vi "2013_01_17 Quality Main.vi"() -> ()   [LabVIEW 2011]
uses:
  <vilib>/DAQmx/write.llb/DAQmx Write (Counter Time 1Chan 1Samp).vi
  <vilib>/DAQmx/read.llb/DAQmx Read (Analog 1D Wfm NChan NSamp).vi
  Quality Type Def.ctl
panel:
  out "position mode":i32
  out "samples available":i32
  in  "Choose Lead":dbl=1.0 min=1.0 max=2.0 step=1.0
  out "XY Graph 2":cluster{"Array":dbl[], "Array":dbl[]}[](graph)
  out "Single Motor 2":waveform(dbl)[](graph)
  in  "Waveform":bool
  out "XY Graph":cluster{"Array":dbl[], "Array":dbl[]}(graph)
  out "error out":errorcluster
  in  "File Path":path=path "Durability/.lvm"
  in  "Motor 1":T1 {"ESC Efficiency" format="%#_3g%%"; "Supply Power (W)" format="%.3g"; "Mechanical Power (W)" format="%.3g"; "Motor Efficiency" format="%#_3g%%"; "Electrical Power (W)" format="%.3g"; "Torque (mNm)" format="%.3g"; "Elapsed Time" format="%<%H:%M:%S>t"; "Supply (V)" format="%.2f"; "RPM" scale=0.0..60000.0}
  out "loop time (ms)":u32
  in  "stop":bool
  in  "PWM 1":dbl(slide) min=0.0 max=100.0 step=5.0 scale=0.0..100.0
  # "Fail"
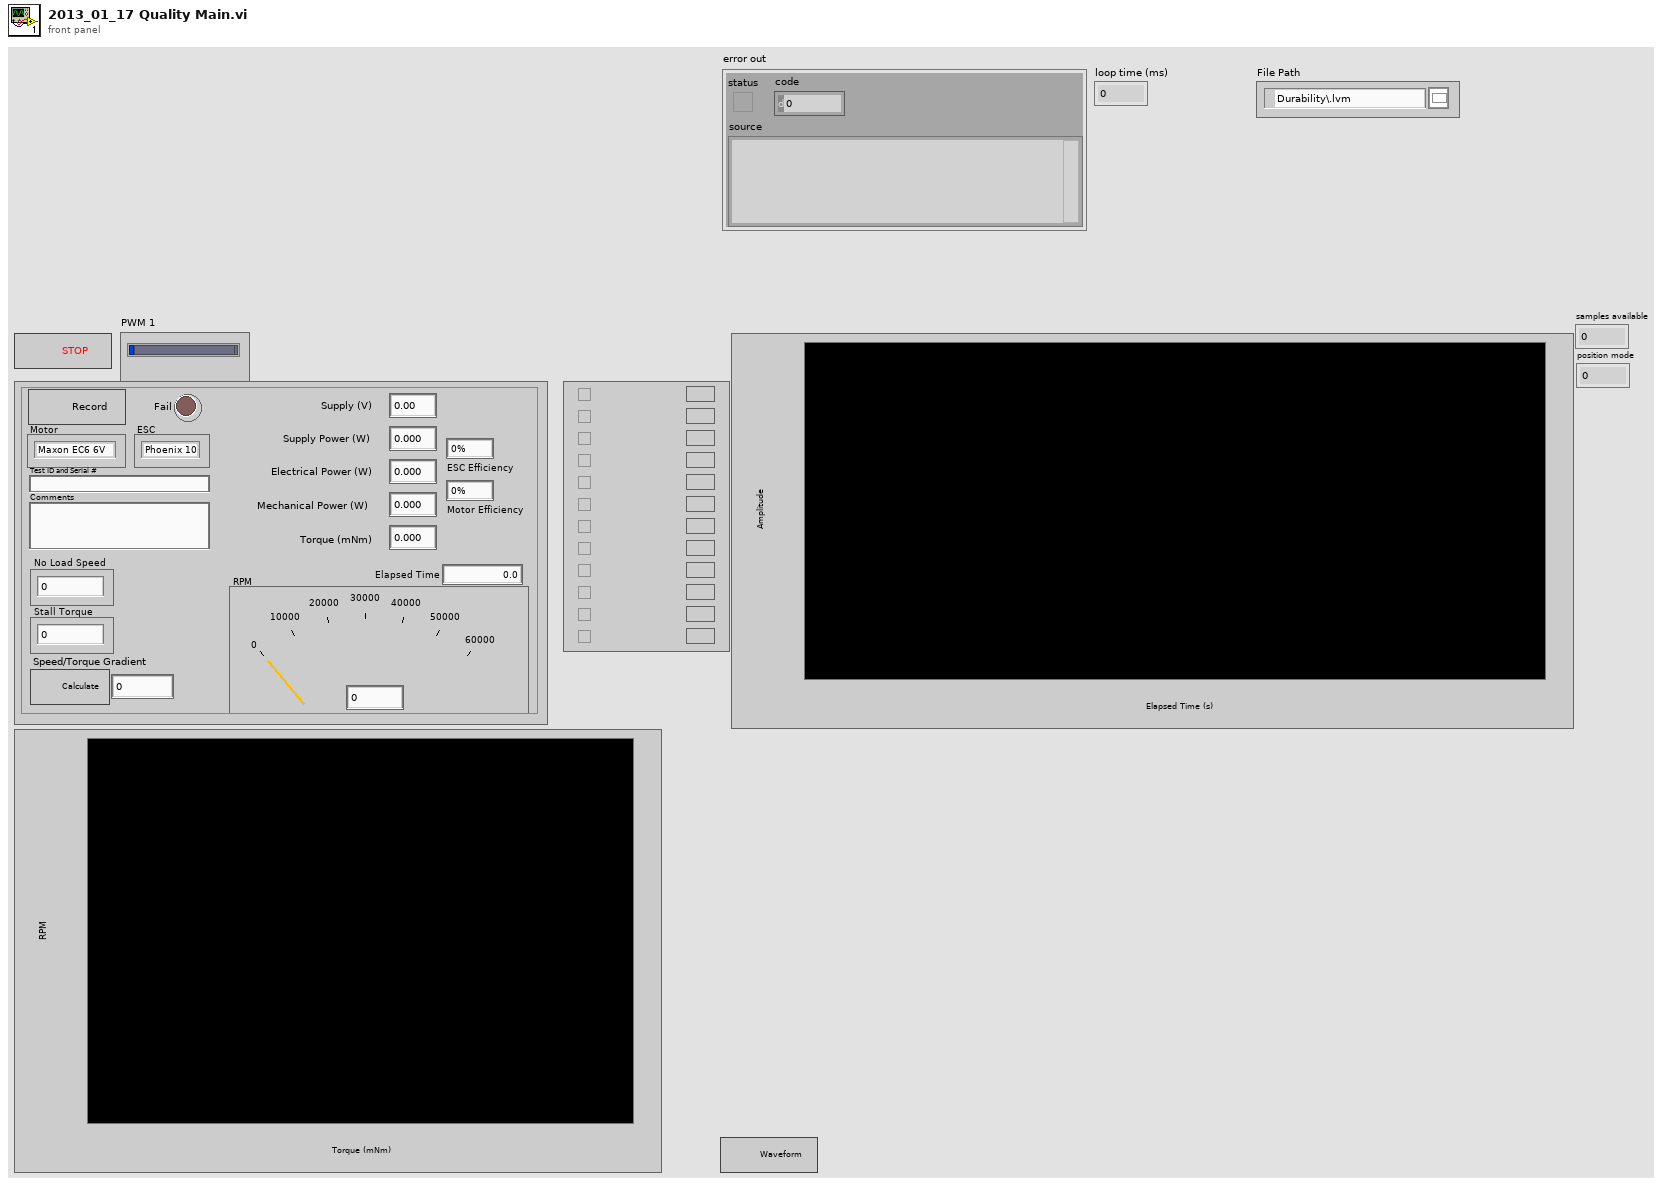
[diagram p1: front panel]
types:
  T1 = typedef "Quality Type Def.ctl" = cluster{"Enabled":bool, "Fail":bool, "RPM":u64, "Motor":enum16{"Maxon EC6 6V", "Maxon EC4 6V", "FH 0620 6V", "FH 0620 12V"}, "ESC":enum16{"Phoenix 10", "Maxon", "FH 1801"}, "Supply (V)":dbl, "Test ID and Serial #":string, "Comments":string, "Elapsed Time":dbl, "Counter":dbl, "Torque (mNm)":dbl, "Electrical Power (W)":dbl, "Motor Efficiency":dbl, "Mechanical Power (W)":dbl, "Supply Power (W)":dbl, "ESC Efficiency":dbl, "No Load Speed":u32, "Stall Torque":dbl, "Speed/Torque Gradient":u32, "Calcul":bool}
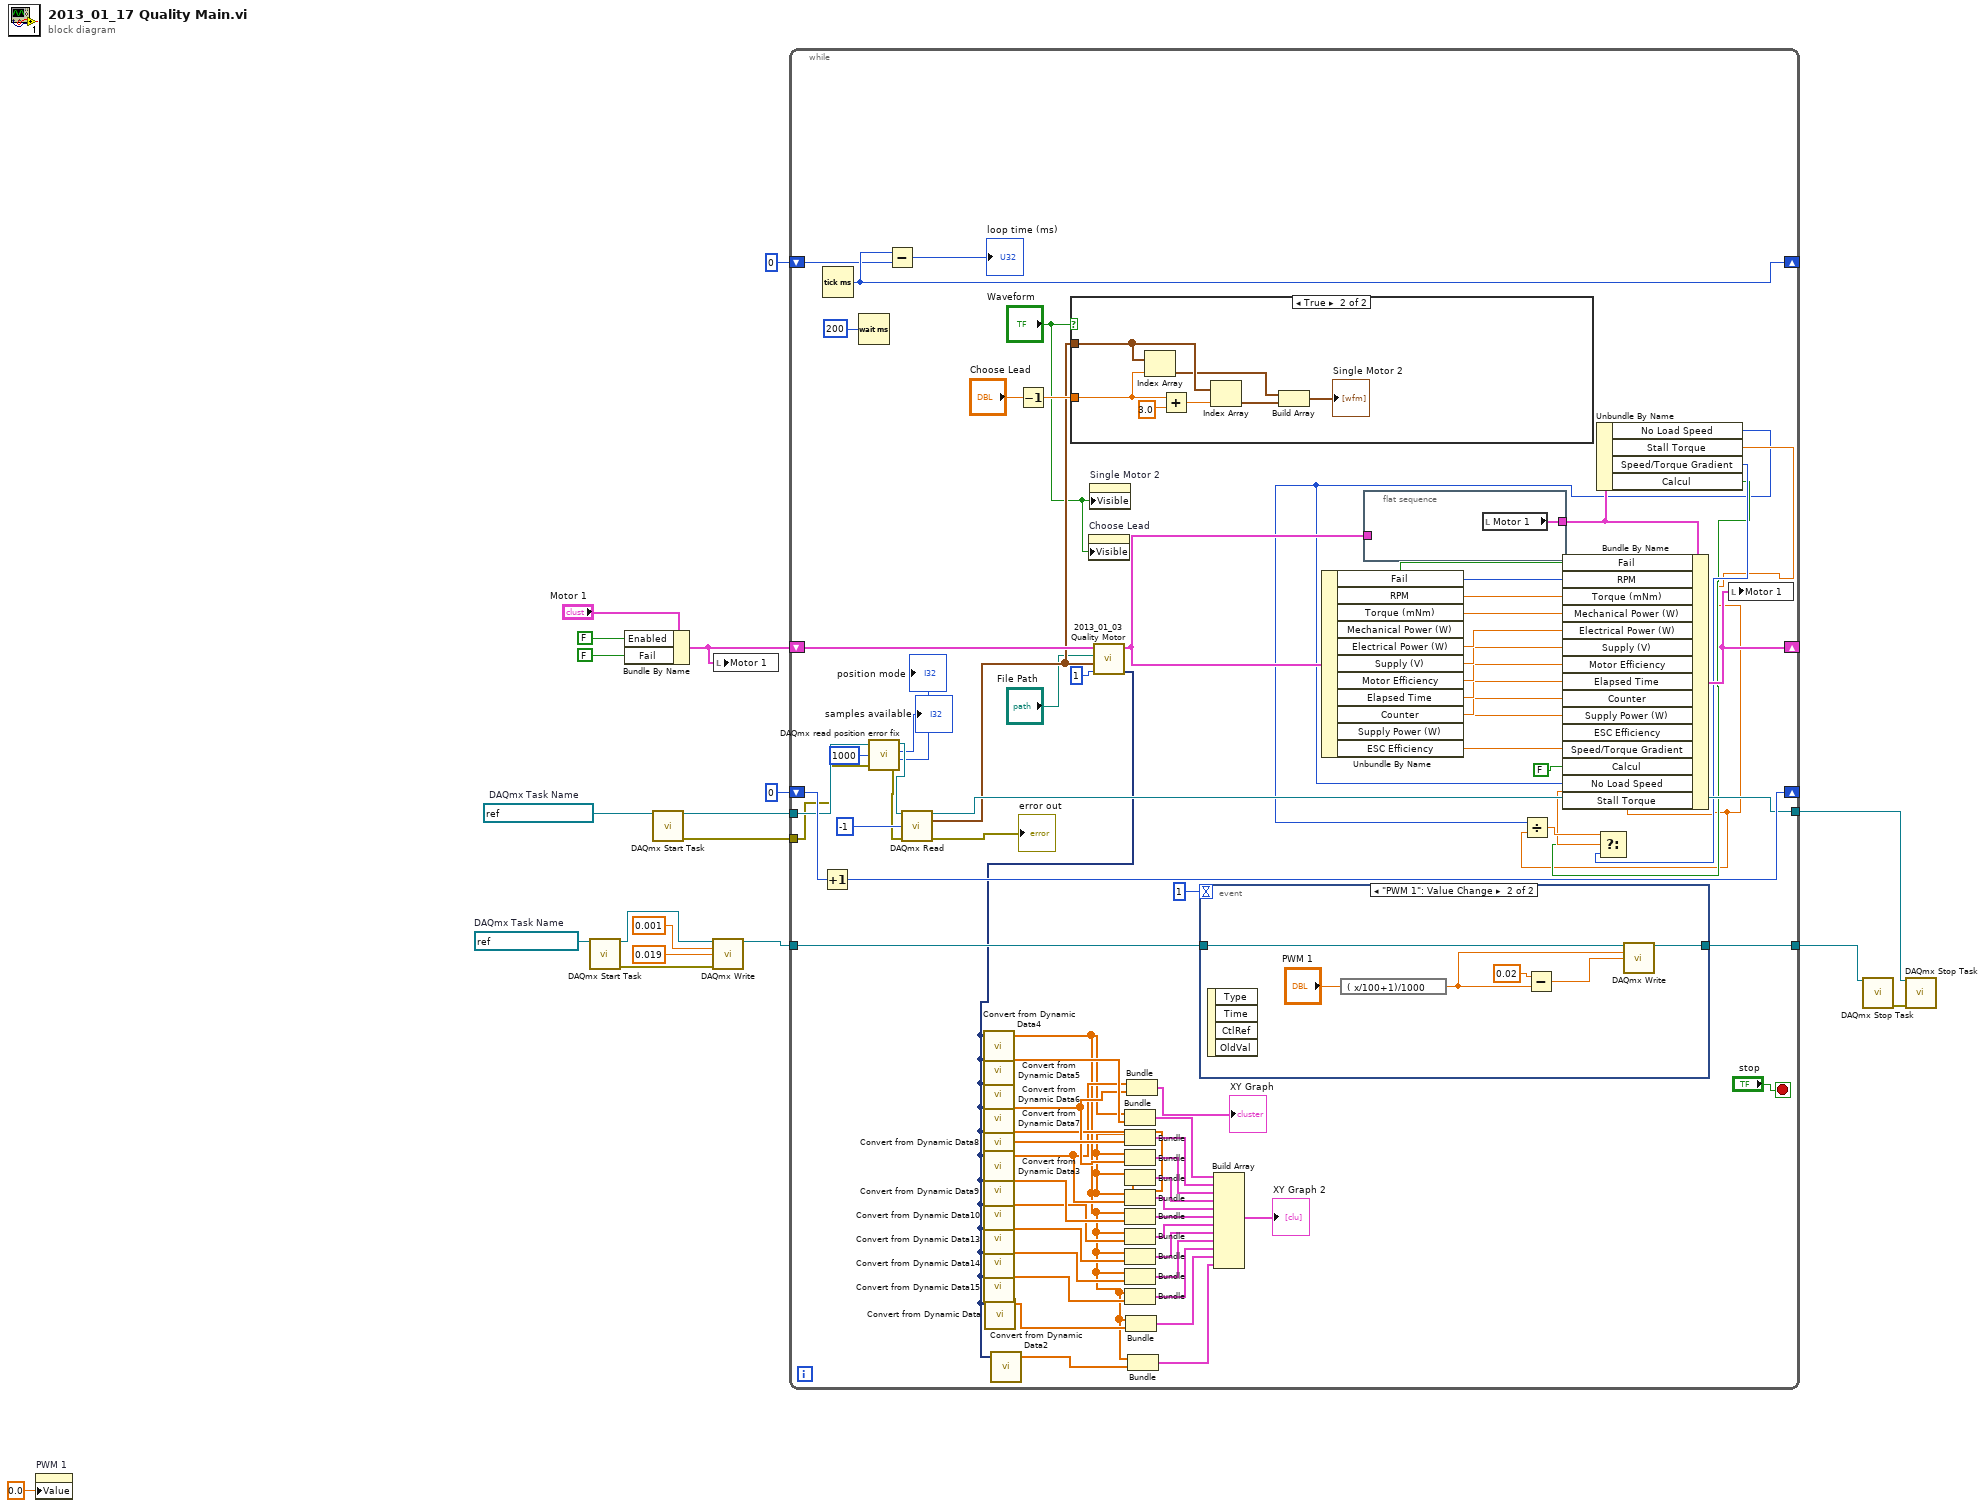
[diagram p0: block diagram]
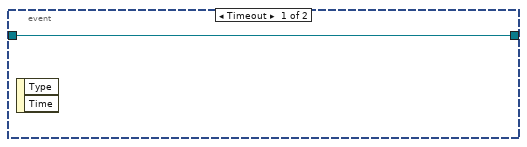
[diagram p3: hidden frame]
diagram:
  w16 = refnum<k21> "Quality PWM1"  # DAQmx Task Name
  w19 = refnum<k21> "Quality Acquire"  # DAQmx Task Name
  n1 = property on="PWM 1" class="Slide (strict)"("Value"=0.0 ("PWM 1")) -> ()  [unwired: 2 in, 2 out]
  n2 = call <vilib>:"DAQmx Start Task.vi"("task/channels in"=w16) -> ("task out"=w14:refnum<k21>, "error out"=w13:errorcluster)  [unwired: 13 in]
  n3 = Bundle By Name(cluster="Motor 1", "Enabled"=FALSE, "Fail"=FALSE) -> (w1:T1)
  n4 = call <vilib>:"DAQmx Start Task.vi"("task/channels in"=w19) -> ("task out"=w18:refnum<k21>, "error out"=w5:errorcluster)  [unwired: 13 in]
  n5 = call-poly <vilib>:"DAQmx Write.vi"("task/channels in"=w14, "high time"=0.001 ("data"), "low time"=0.019 ("data"), "error in"=w13) -> ("task out"=w15:refnum<k21>)  [unwired: 9 in, 2 out]
  n6 = local write "Motor 1"(w1) -> ()
  n7 = while {
    tunnel: w18 -> [w26]
    tunnel: [w82] -> w17
    tunnel: w5 -> [w24]
    shift-right: [w94] -> _
    shift-left: u32 0 ("millisecond timer value") -> [w93]
    tunnel: w15 -> [w91]
    tunnel: [w90] -> w12
    shift-right: [w72] -> _
    shift-left: w1 -> [w71]
    shift-right: [w87] -> _
    shift-left: 0 ("for") -> [w88]
    stop <- "stop" stop-if-true
    n8 = Increment(x=w88) -> (x+1=w87:i32)
    n9 = Tick Count (ms)() -> (millisecond timer value=w94:u32)
    n10 = Wait (ms)(milliseconds to wait=u32 200) -> ()  [unwired: 1 out]
    n11 = call "DAQmx read position error fix.vi"("task in"=w26, "samples to read"=1000, "error in"=w24) -> ("task out"=w25:refnum<k21>, "samples available"=→"samples available":i32, "position mode"=→"position mode":i32, "error out"=w23:errorcluster)
    n12 = Subtract(x=w94, y=w93) -> (x-y=→"loop time (ms)":u32)
    n13 = call-poly <vilib>:"DAQmx Read.vi"("task/channels in"=w25, "number of samples per channel"=-1, "error in"=w23) -> ("task out"=w82:refnum<k21>, "data"=w68:waveform(dbl)[], "error out"=→"error out":errorcluster)  [unwired: 10 in]
    n14 = Decrement(x="Choose Lead") -> (x-1=w83:dbl)
    n15 = case shown="True" "Waveform" {
      tunnel: w68 -> [_ w100]
      tunnel: w83 -> [_ w101]
      frame False {
      }
      frame True {
        n16 = Index Array(array=w100, index=w101) -> (element=w98:waveform(dbl))
        n17 = Add(x=w101, y=3.0) -> (x+y=w99:dbl)
        n18 = Index Array(array=w100, index=w99) -> (element=w97:waveform(dbl))
        n19 = Build Array(w98, w97) -> (→"Single Motor 2":waveform(dbl)[])
      }
    }
    n20 = property on="Choose Lead" class="DigNum (strict)"("Visible"="Waveform") -> ()  [unwired: 2 in, 2 out]
    n21 = property on="Single Motor 2" class="WFGraph (strict)"("Visible"="Waveform") -> ()  [unwired: 2 in, 2 out]
    n22 = call "2013_01_03 Quality Motor.vi"("Motor #"=1, "data"=w68, "File Path"="File Path", "Motor Typedef"=w71) -> ("Final Out"=w39:dynamicdata, "Motor Typedef Out"=w70:T1)  [unwired: 6 in]
    n23 = call "Convert from Dynamic Data4"("Dynamic Data Type"=w39) -> ("Array"=w41:dbl[])  [unwired: 3 in]
    n24 = call "Convert from Dynamic Data5"("Dynamic Data Type"=w39) -> ("Array"=w55:dbl[])  [unwired: 3 in]
    n25 = call "Convert from Dynamic Data6"("Dynamic Data Type"=w39) -> ("Array"=w54:dbl[])  [unwired: 3 in]
    n26 = call "Convert from Dynamic Data7"("Dynamic Data Type"=w39) -> ("Array"=w53:dbl[])  [unwired: 3 in]
    n27 = call "Convert from Dynamic Data8"("Dynamic Data Type"=w39) -> ("Array"=w52:dbl[])  [unwired: 3 in]
    n28 = call "Convert from Dynamic Data3"("Dynamic Data Type"=w39) -> ("Array"=w51:dbl[])  [unwired: 3 in]
    n29 = call "Convert from Dynamic Data9"("Dynamic Data Type"=w39) -> ("Array"=w50:dbl[])  [unwired: 3 in]
    n30 = call "Convert from Dynamic Data10"("Dynamic Data Type"=w39) -> ("Array"=w49:dbl[])  [unwired: 3 in]
    n31 = call "Convert from Dynamic Data13"("Dynamic Data Type"=w39) -> ("Array"=w48:dbl[])  [unwired: 3 in]
    n32 = call "Convert from Dynamic Data14"("Dynamic Data Type"=w39) -> ("Array"=w47:dbl[])  [unwired: 3 in]
    n33 = call "Convert from Dynamic Data15"("Dynamic Data Type"=w39) -> ("Array"=w46:dbl[])  [unwired: 3 in]
    n34 = call "Convert from Dynamic Data"("Dynamic Data Type"=w39) -> ("Array"=w43:dbl[])  [unwired: 3 in]
    n35 = call "Convert from Dynamic Data2"("Dynamic Data Type"=w39) -> ("Array"=w40:dbl[])  [unwired: 3 in]
    n36 = Bundle("Array"=w41, "Array"=w55) -> (w56:cluster{"Array":dbl[], "Array":dbl[]})  [unwired: 1 in]
    n37 = Bundle("Array"=w41, "Array"=w54) -> (w57:cluster{"Array":dbl[], "Array":dbl[]})  [unwired: 1 in]
    n38 = Bundle("Array"=w41, "Array"=w53) -> (w58:cluster{"Array":dbl[], "Array":dbl[]})  [unwired: 1 in]
    n39 = Bundle("Array"=w41, "Array"=w52) -> (w59:cluster{"Array":dbl[], "Array":dbl[]})  [unwired: 1 in]
    n40 = Bundle("Array"=w41, "Array"=w51) -> (w60:cluster{"Array":dbl[], "Array":dbl[]})  [unwired: 1 in]
    n41 = Bundle("Array"=w41, "Array"=w50) -> (w61:cluster{"Array":dbl[], "Array":dbl[]})  [unwired: 1 in]
    n42 = Bundle("Array"=w41, "Array"=w49) -> (w62:cluster{"Array":dbl[], "Array":dbl[]})  [unwired: 1 in]
    n43 = Bundle("Array"=w41, "Array"=w48) -> (w63:cluster{"Array":dbl[], "Array":dbl[]})  [unwired: 1 in]
    n44 = Bundle("Array"=w41, "Array"=w47) -> (w65:cluster{"Array":dbl[], "Array":dbl[]})  [unwired: 1 in]
    n45 = Bundle("Array"=w41, "Array"=w46) -> (w64:cluster{"Array":dbl[], "Array":dbl[]})  [unwired: 1 in]
    n46 = Bundle("Array"=w41, "Array"=w43) -> (w42:cluster{"Array":dbl[], "Array":dbl[]})  [unwired: 1 in]
    n47 = Bundle("Array"=w51, "Array"=w53) -> (→"XY Graph":cluster{"Array":dbl[], "Array":dbl[]})  [unwired: 1 in]
    n48 = Bundle("Array"=w41, "Array"=w40) -> (w38:cluster{"Array":dbl[], "Array":dbl[]})  [unwired: 1 in]
    n49 = event shown="[1] \"PWM 1\": Value Change" {
      selector: _ -> [_ _]
      dyn-events: _ -> [_ _]
      timeout: 1 -> [_ _]
      tunnel: w91 -> [w104 w106]
      tunnel: [w104 w105] -> w90
      event Timeout {
        n50 = event-data() -> ()  [unwired: 1 in, 2 out]
      }
      event "PWM 1": Value Change {
        n51 = event-data() -> ()  [unwired: 1 in, 4 out]
        n52 = expression code="( x/100+1)/1000"("PWM 1") -> (w107:dbl)
        n53 = Subtract(x=0.02 ("y"), y=w107) -> (x-y=w108:dbl)
        n54 = call-poly <vilib>:"DAQmx Write.vi"("task/channels in"=w106, "high time"=w107, "low time"=w108) -> ("task out"=w105:refnum<k21>)  [unwired: 10 in, 2 out]
      }
    }
    n55 = Build Array(w56, w57, w58, w59, w60, w61, w62, w63, w65, w64, w42, w38) -> (→"XY Graph 2":cluster{"Array":dbl[], "Array":dbl[]}[])
    n56 = Unbundle By Name(w70) -> ("Fail"=w81:bool, "RPM"=w80:u64, "Torque (mNm)"=w79:dbl, "Mechanical Power (W)"=w78:dbl, "Electrical Power (W)"=w77:dbl, "Supply (V)"=w76:dbl, "Motor Efficiency"=w75:dbl, "Elapsed Time"=w74:dbl, "Counter"=w73:dbl, "Supply Power (W)"=w36:dbl, "ESC Efficiency"=w37:dbl)
    n57 = flat-sequence {
      tunnel: w70 -> [_]
      tunnel: [w103] -> w32
      frame #0 {
        n58 = local read "Motor 1"() -> (w103:T1)
      }
    }
    n59 = Unbundle By Name(w32) -> ("No Load Speed"=w28:u32, "Stall Torque"=w29:dbl, "Speed/Torque Gradient"=w31:u32, "Calcul"=w30:bool)
    n60 = Divide(x=w28, y=w29) -> (x/y=w34:dbl)
    n61 = Select(t=w34, s=w30, f=w31) -> (s? t:f=w33:dbl)
    n62 = Bundle By Name(cluster=w32, "Fail"=w81, "RPM"=w80, "Torque (mNm)"=w79, "Mechanical Power (W)"=w78, "Electrical Power (W)"=w77, "Supply (V)"=w76, "Motor Efficiency"=w75, "Elapsed Time"=w74, "Counter"=w73, "Supply Power (W)"=w36, "ESC Efficiency"=w37, "Speed/Torque Gradient"=w33, "Calcul"=FALSE, "No Load Speed"=w28, "Stall Torque"=w29) -> (w72:T1)
    n63 = local write "Motor 1"(w72) -> ()
  }
  n64 = call <vilib>:"DAQmx Stop Task.vi"("task/channels in"=w12) -> ("error out"=w11:errorcluster)  [unwired: 13 in, 1 out]
  n65 = call <vilib>:"DAQmx Stop Task.vi"("task/channels in"=w17, "error in"=w11) -> ()  [unwired: 12 in, 2 out]
